vi "FieldDisp_Field_Selector_Prepare.vi"(11 "ComboBox Ref":refnum<vi>) -> (0 "error out":errorcluster, 3 "section names":string[](array[string]))   [LabVIEW 2019, in "Trajectory_Library.lvlib"]
doc: "Read the field information INI file and update a ComboBox control with the list of available fields.\n\nThe field information INI file must be in a FieldInfo subdirectory under the application's main directory. The field image files are also located in this subdirectory.\n\nInputs:\n - ComboBox Ref -- ComboBox Control Reference -- Reference to the control to be updated.\n\nOutputs:\n - Section Names -- String array -- List of field names.\n - Error out -- error cluster -- If an error occured, contains error information."
uses:
  Trajectory_Library.lvlib
  <vilib>/Utility/config.llb/NI_LVConfig.lvlib
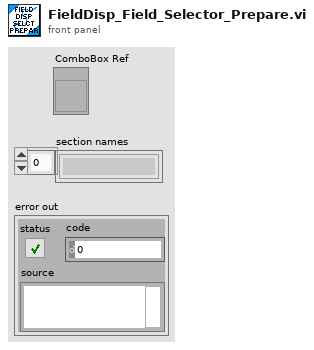
[diagram p1: front panel]
types:
  T1 = typedef "NI_LVConfig.lvlib/Config Data RefNum.ctl" = refnum<k1>
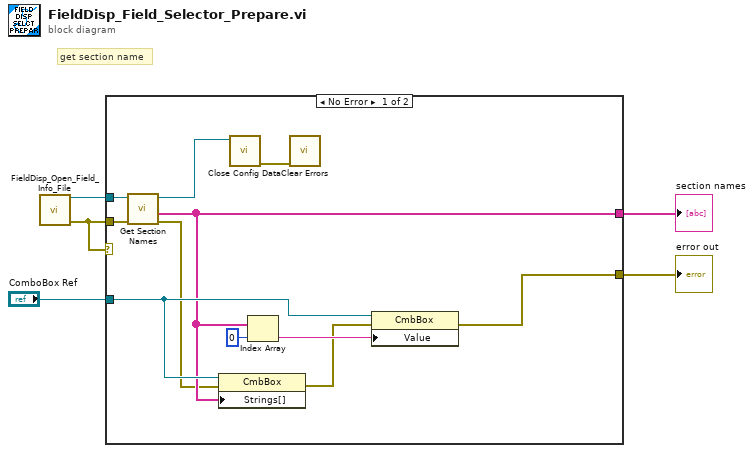
[diagram p0: block diagram]
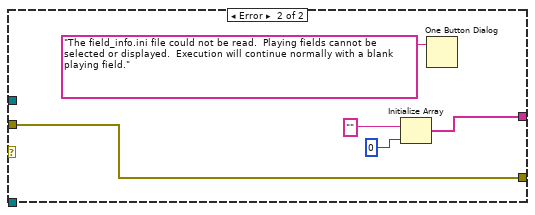
[diagram p2: hidden frame]
diagram:
  # "get section name"
  n1 = call "FieldDisp_Open_Field_Info_File.vi"() -> ("error out"=w2:errorcluster, "Refnum out"=w3:T1)  [unwired: 10 in]
  n2 = case shown="No Error" w2 {
    tunnel: [w6 w21] -> w5
    tunnel: w2 -> [w15 w21]
    tunnel: [w8 w17] -> w4
    tunnel: w3 -> [w14 _]
    tunnel: "ComboBox Ref" -> [w9 _]
    frame No Error {
      n3 = call <vilib>:"Get Section Names.vi"("error in (no error)"=w15, "refnum"=w14) -> ("error out"=w7:errorcluster, "section names"=w8:string[], "refnum out"=w16:T1)  [unwired: 7 in]
      n4 = property on="Property Node" class="CmbBox"(reference=w9, error in=w7, "Strings[]"=w8) -> (error out=w10:errorcluster)  [unwired: 1 out]
      n5 = call <vilib>:"Close Config Data.vi"("refnum"=w16) -> ("error out"=w13:errorcluster)  [unwired: 9 in, 1 out]
      n6 = Index Array(array=w8, index=0) -> (element=w11:string)
      n7 = call <vilib>:"Clear Errors.vi"("error in (no error)"=w13) -> ()  [unwired: 5 in, 2 out]
      n8 = property on="Property Node" class="CmbBox"(reference=w9, error in=w10, "Value"=w11) -> (error out=w6:errorcluster)  [unwired: 1 out]
    }
    frame Error {
      n9 = Initialize Array("" ("String"), 0 ("dimension size")) -> (w17:string[])
      n10 = One Button Dialog(message="The field_info.ini file could not be read.  Playing fields cannot be selected or displayed.  Execution will continue normally with a blank playing field.") -> ()  [unwired: 1 in, 1 out]
    }
  }
  "error out" <- w5
  "section names" <- w4
